vi "Build Trigger Terminal.vi"(8 "error in (no error)":errorcluster, 9 "Trigger/Event Name":string(combo)="SourceTrigger", 10 "Channel Name":string="0", 11 "Resource Name":string) -> (0 "error out":errorcluster, 3 "Terminal Name":string)   [LabVIEW 2021]
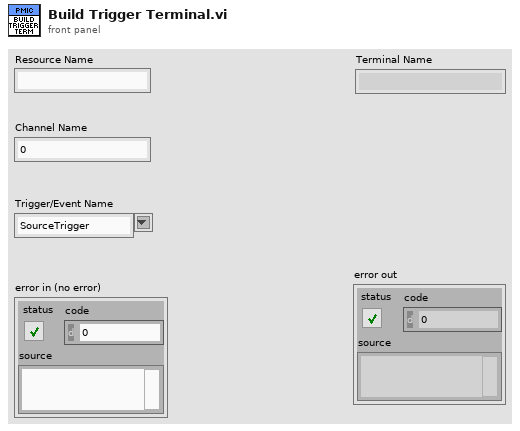
[diagram p1: front panel]
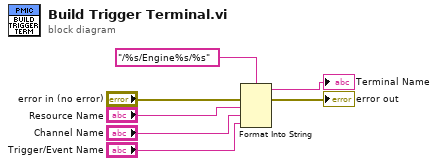
[diagram p0: block diagram]
diagram:
  n1 = Format Into String(format string="/%s/Engine%s/%s", error in="error in (no error)", "Resource Name", "Channel Name", "Trigger/Event Name") -> (resulting string=→"Terminal Name":string, error out=→"error out":errorcluster)  [unwired: 1 in]
